vi "CloseLabVIEW.vi"   [LabVIEW 2014]
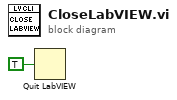
[diagram p0: block diagram]
diagram:
  n1 = Quit LabVIEW(quit? (T)=TRUE) -> ()
